vi "Quest Sub Register.vi"(8 "error in (no error)":errorcluster, 9 "Sub Register(0:Quest Enable Register)":u16(ring) items=["Quest Enable Register?", "Quest Status register?", "Quest Event Register?"], 10 "Channel Select":enum16{"Channel 1", "Channel 2", "Channel 3"}(ring), 11 "Visa Resource Name IN":refnum<visa-resource-name>) -> (0 "error out":errorcluster, 2 "Sub Register Response":string, 3 "Visa Resource Name OUT":refnum<visa-resource-name>)   [LabVIEW 2018, in "Keithley KE22xx Series.lvlib"]
doc: "Display the status of different Quest Sub Register for specified channel.\n\nQuest Sub Registers:\n1.Quest Enable Register\n2.Quest Status Register\n3.Quest Event Register"
uses:
  Keithley KE22xx Series.lvlib
panel:
  # "© 2012 Keithley Instruments, Inc. ALL RIGHTS RESERVED"
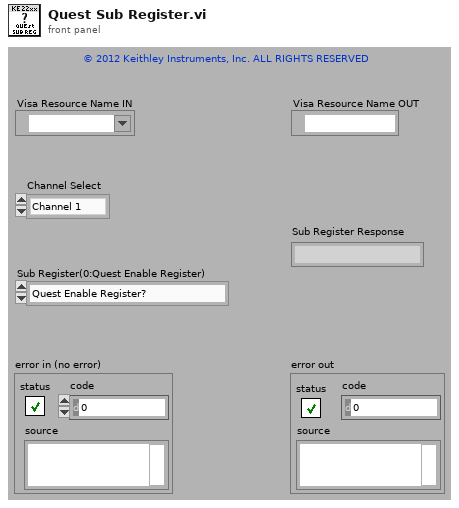
[diagram p1: front panel]
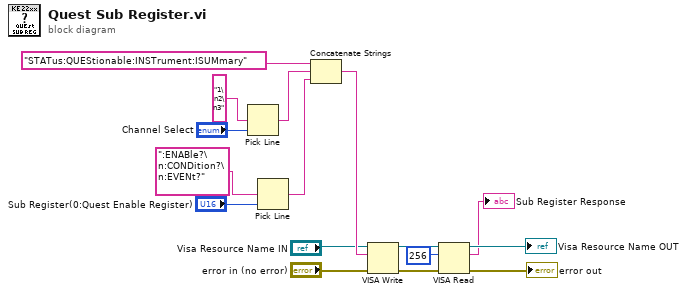
[diagram p0: block diagram]
diagram:
  n1 = Pick Line(multi-line string="1\n2\n3", line index="Channel Select") -> (output string=w13:string)  [unwired: 1 in]
  n2 = Pick Line(multi-line string=":ENABle?\n:CONDition?\n:EVENt?", line index="Sub Register(0:Quest Enable Register)") -> (output string=w1:string)  [unwired: 1 in]
  n3 = Concatenate Strings("STATus:QUEStionable:INSTrument:ISUMmary", w13, w1) -> (w12:string)
  n4 = VISA Write(VISA resource name="Visa Resource Name IN", write buffer=w12, error in (no error)="error in (no error)") -> (VISA resource name out=w11:refnum<visa-resource-name>, error out=w10:errorcluster)  [unwired: 1 out]
  n5 = VISA Read(VISA resource name=w11, byte count=u32 256, error in (no error)=w10) -> (VISA resource name out=→"Visa Resource Name OUT":refnum<visa-resource-name>, read buffer=→"Sub Register Response":string, error out=→"error out":errorcluster)  [unwired: 1 out]
